vi "设置.vi"() -> ()   [LabVIEW 2016, in "数据查询.lvlib"]
uses:
  <vilib>/Utility/miscctls.llb/LVPointTypeDef.ctl
  var/holding var.vi
panel:
  out "字符串":string
  in  "数据库备份位置":path
  in  "重建数据表":bool
  in  "自动备份":bool
  in  "备份周期":enum16{"每小时", "每天", "每周", "每月"}(ring)
  # "数据库自动备份："
  # "数据库备份周期："
  # "数据库备份路径："
  # "重建数据表："
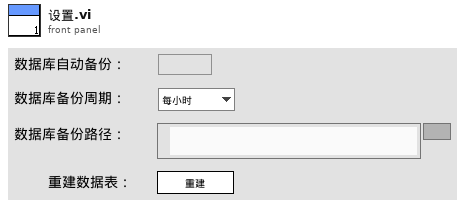
[diagram p1: front panel]
types:
  T1 = typedef "LVPointTypeDef.ctl" = cluster{"Horizontal":i16, "Vertical":i16}
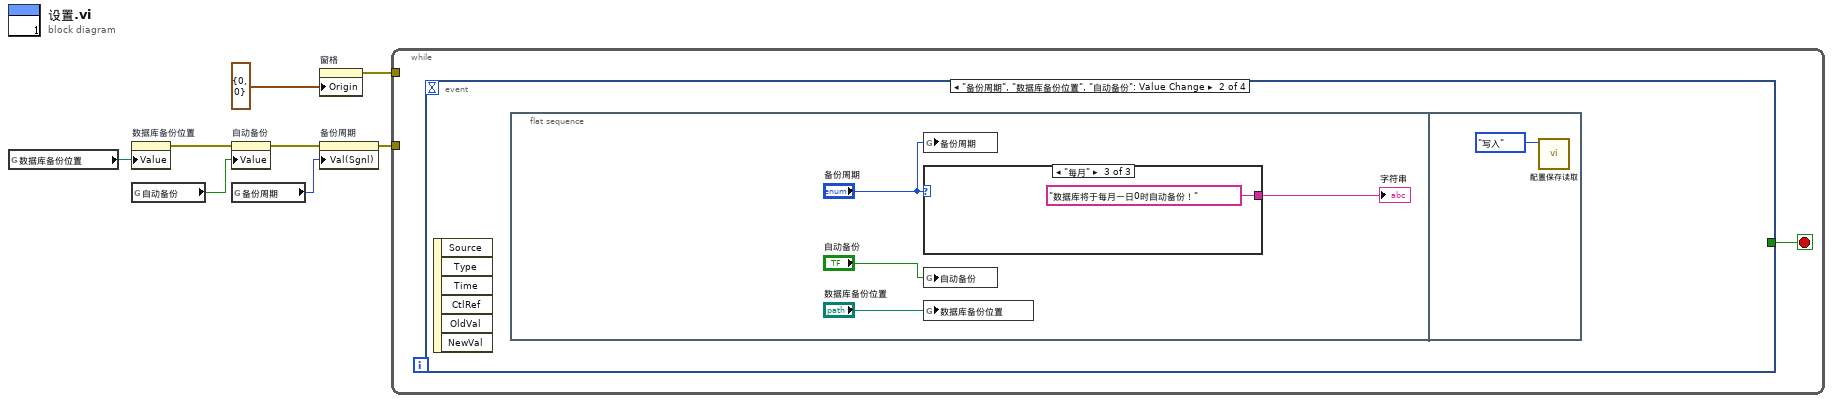
[diagram p0: block diagram]
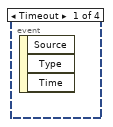
[diagram p2: hidden frame]
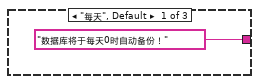
[diagram p3: hidden frame]
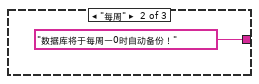
[diagram p4: hidden frame]
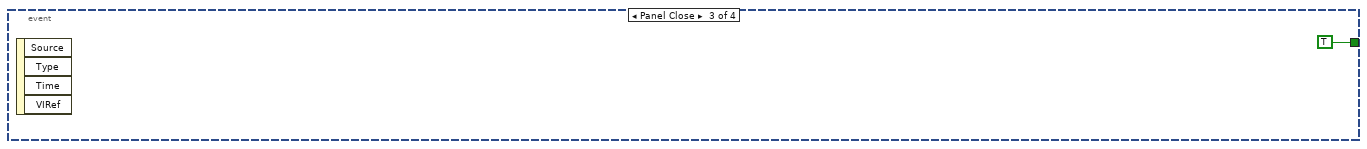
[diagram p5: hidden frame]
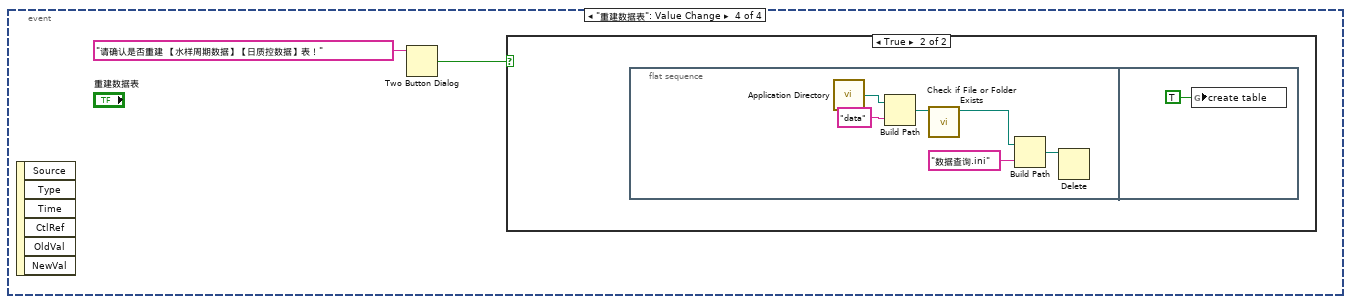
[diagram p6: hidden frame]
diagram:
  n1 = global read "holding var.vi" "数据库备份位置"() -> (w5:path)
  n2 = property on="数据库备份位置" class="Path"("Value"=w5) -> (error out=w6:errorcluster)  [unwired: 2 in, 1 out]
  n3 = global read "holding var.vi" "自动备份"() -> (w4:bool)
  n4 = property on="自动备份" class="Bool (strict)"(error in=w6, "Value"=w4) -> (error out=w2:errorcluster)  [unwired: 1 in, 1 out]
  n5 = global read "holding var.vi" "备份周期"() -> (w3:enum16{"每小时", "每天", "每周", "每月"})
  n6 = property on="窗格" class="Pane"("Origin"=T1 {"Horizontal"=0, "Vertical"=0} ("原点")) -> (error out=w7:errorcluster)  [unwired: 2 in, 1 out]
  n7 = property on="备份周期" class="Enum (strict)"(error in=w2, "Val(Sgnl)"=w3) -> (error out=w1:errorcluster)  [unwired: 1 in, 1 out]
  n8 = while {
    tunnel: w7 -> [_]
    tunnel: w1 -> [_]
    stop <- w9 stop-if-true
    n9 = event shown="[1] \"备份周期\", \"数据库备份位置\", \"自动备份\": Value Change" {
      selector: _ -> [_ _ _ _]
      dyn-events: _ -> [_ _ _ _]
      timeout: _ -> [_ _ _ _]
      tunnel: [_ _ TRUE _] -> w9
      event Timeout {
        n10 = event-data() -> ()  [unwired: 1 in, 3 out]
      }
      event "备份周期", "数据库备份位置", "自动备份": Value Change {
        n11 = event-data() -> ()  [unwired: 1 in, 6 out]
        n12 = flat-sequence {
          frame #0 {
            n13 = global write "holding var.vi" "备份周期"("备份周期") -> ()
            n14 = case shown="\"每月\"" "备份周期" {
              tunnel: ["数据库将于每天0时自动备份！" ("字符串") "数据库将于每周一0时自动备份！" ("字符串") "数据库将于每月一日0时自动备份！" ("字符串")] -> w11
              frame "每天", Default {
              }
              frame "每周" {
              }
              frame "每月" {
              }
            }
            "字符串" <- w11
            n15 = global write "holding var.vi" "自动备份"("自动备份") -> ()
            n16 = global write "holding var.vi" "数据库备份位置"("数据库备份位置") -> ()
          }
          frame #1 {
            n17 = call "配置保存读取.vi"("配置"=enum16{"读取", "写入"}."写入") -> ()  [unwired: 10 in, 1 out]
          }
        }
      }
      event Panel Close {
        n18 = event-data() -> ()  [unwired: 1 in, 4 out]
      }
      event "重建数据表": Value Change {
        n19 = event-data() -> ()  [unwired: 1 in, 6 out]
        n20 = Two Button Dialog(message="请确认是否重建 【水样周期数据】【日质控数据】表！" ("消息")) -> (T button?=w20:bool)  [unwired: 2 in]
        n21 = case shown="True" w20 {
          frame False {
          }
          frame True {
            n22 = flat-sequence {
              frame #0 {
                n23 = call <vilib>:"Application Directory.vi"() -> ("Application Directory"=w25:path)
                n24 = Build Path(base path=w25, name or relative path="data" ("名称或相对路径")) -> (appended path=w23:path)
                n25 = call <vilib>:"Check if File or Folder Exists.vi"("path"=w23) -> ("dup path"=w22:path)  [unwired: 8 in, 2 out]
                n26 = Build Path(base path=w22, name or relative path="数据查询.ini" ("名称或相对路径")) -> (appended path=w26:path)
                n27 = Delete(path (use dialog)=w26) -> ()  [unwired: 4 in, 3 out]
              }
              frame #1 {
                n28 = global write "全局变量.vi" "create table"(TRUE ("create table")) -> ()
              }
            }
          }
        }
      }
    }
  }
